vi "YokoGS200 Set Limits.vi"(6 "Set Limit":enum16{"Current", "Voltage", "Both"}(ring), 8 "error in (no error)":errorcluster, 9 "VoltLimit":dbl=1.0 caption="Voltage Limit" min=1.0 max=30.0 step=1.0, 10 "CurrLimit":dbl=0.001 caption="Current Limit" min=0.001 max=0.2 step=0.001, 11 "VISA Rsrc":refnum<visa-resource-name>="SR530") -> (0 "error out":errorcluster, 1 "VoltLimit 2":dbl caption="Voltage Limit", 2 "CurrLimit Out":dbl caption="Current Limit", 3 "VISA Rsrc Out":refnum<visa-resource-name>="GPIB0::12::INSTR", 4 "ChaineCom":string caption="Chaîne de commande")   [LabVIEW 2019]
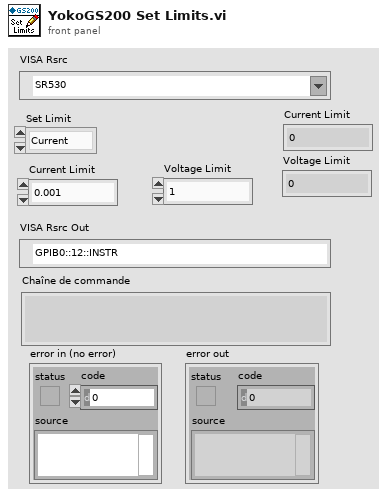
[diagram p1: front panel]
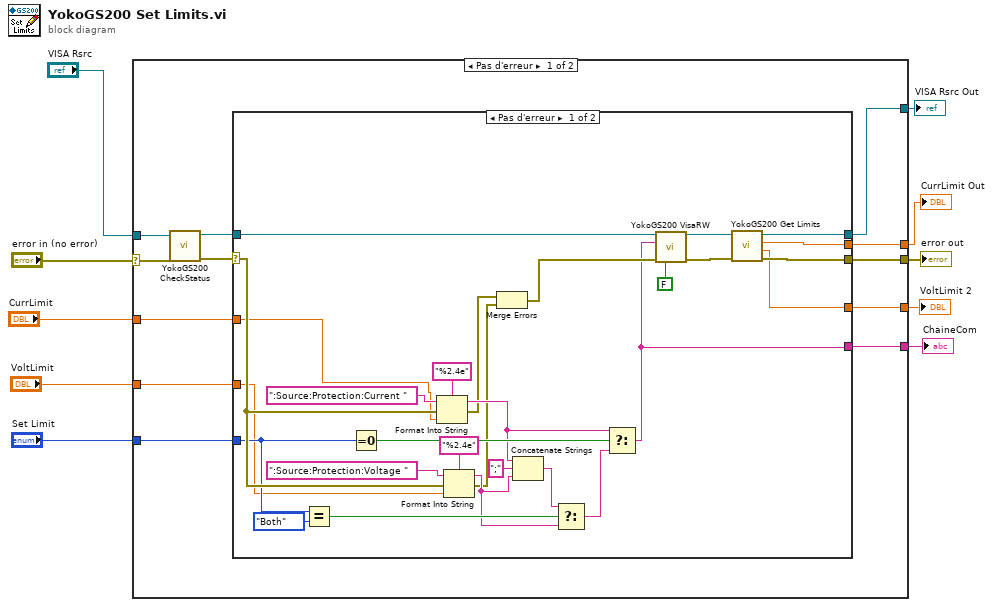
[diagram p0: block diagram]
diagram:
  n1 = case shown="Pas d'erreur" "error in (no error)" {
    selector: "error in (no error)" -> [w19 w53]
    tunnel: "VISA Rsrc" -> [w20 w54]
    tunnel: [w21 w53] -> w8
    tunnel: [w22 w54] -> w7
    tunnel: "Set Limit" -> [w14 _]
    tunnel: "CurrLimit" -> [w16 _]
    tunnel: "VoltLimit" -> [w15 _]
    tunnel: [w13 _] -> w3
    tunnel: [w12 _] -> w2
    tunnel: [w11 _] -> w1
    frame No Error {
      n2 = call <userlib>:"YokoGS200 CheckStatus.vi"("error in (no error)"=w19, "VISA Rsrc"=w20) -> ("error out"=w18:errorcluster, "VISA Rsrc Out"=w17:refnum<visa-resource-name>)  [unwired: 6 in, 2 out]
      n3 = case shown="Pas d'erreur" w18 {
        selector: w18 -> [w43 w51]
        tunnel: [w25 w52] -> w22
        tunnel: [w26 w51] -> w21
        tunnel: w17 -> [w49 w52]
        tunnel: w16 -> [w31 _]
        tunnel: w15 -> [w30 _]
        tunnel: w14 -> [w42 _]
        tunnel: [w29 _] -> w13
        tunnel: [w24 _] -> w12
        tunnel: [w23 _] -> w11
        frame No Error {
          n4 = Equal?(x=w42, y=enum16{"Current", "Voltage", "Both"}."Both") -> (x = y?=w40:bool)
          n5 = Equal To 0?(x=w42) -> (x = 0?=w44:bool)
          n6 = Format Into String(format string="%2.4e", initial string=":Source:Protection:Current " ("string (\"\")"), error in=w43, w31) -> (resulting string=w37:string, error out=w33:errorcluster)
          n7 = Format Into String(format string="%2.4e", initial string=":Source:Protection:Voltage " ("string (\"\")"), error in=w43, w30) -> (resulting string=w36:string, error out=w34:errorcluster)
          n8 = Merge Errors(w33, w34) -> (w32:errorcluster)
          n9 = Concatenate Strings(w37, ";" ("string"), w36) -> (w35:string)
          n10 = Select(t=w35, s=w40, f=w36) -> (s? t:f=w39:string)
          n11 = Select(t=w37, s=w44, f=w39) -> (s? t:f=w29:string)
          n12 = call <userlib>:"YokoGS200 VisaRW.vi"("VISA Rsrc"=w49, "ChaineCom"=w29, "error in (no error)"=w32, "Lecture?(T)"=FALSE) -> ("VISA Rsrc Out"=w27:refnum<visa-resource-name>, "error out"=w28:errorcluster)  [unwired: 7 in, 3 out]
          n13 = call <userlib>:"YokoGS200 Get Limits.vi"("error in (no error)"=w28, "VISA Rsrc"=w27) -> ("error out"=w26:errorcluster, "VoltLimit"=w23:dbl, "CurrLimit"=w24:dbl, "VISA Rsrc Out"=w25:refnum<visa-resource-name>)  [unwired: 6 in]
        }
        frame Error {
        }
      }
    }
    frame Error {
    }
  }
  "error out" <- w8
  "VISA Rsrc Out" <- w7
  "ChaineCom" <- w3
  "CurrLimit Out" <- w2
  "VoltLimit 2" <- w1
